vi "Lab 7.vi"() -> ()   [LabVIEW 2021]
uses:
  <vilib>/Utility/file.llb/Write Delimited Spreadsheet (string).vi
panel:
  in  "Delete User":bool
  in  "Add User":bool
  in  "Login":bool
  in  "Table Control":string[][](table)
  out "?":bool
  in  "Password:":string
  in  "Username:":string
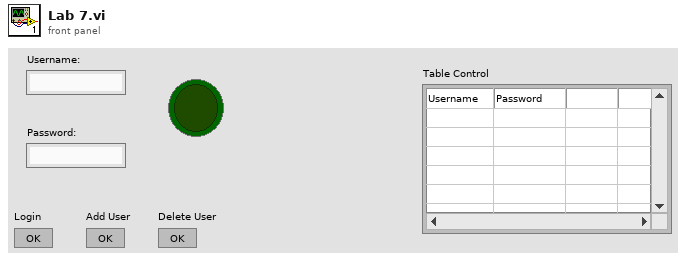
[diagram p1: front panel]
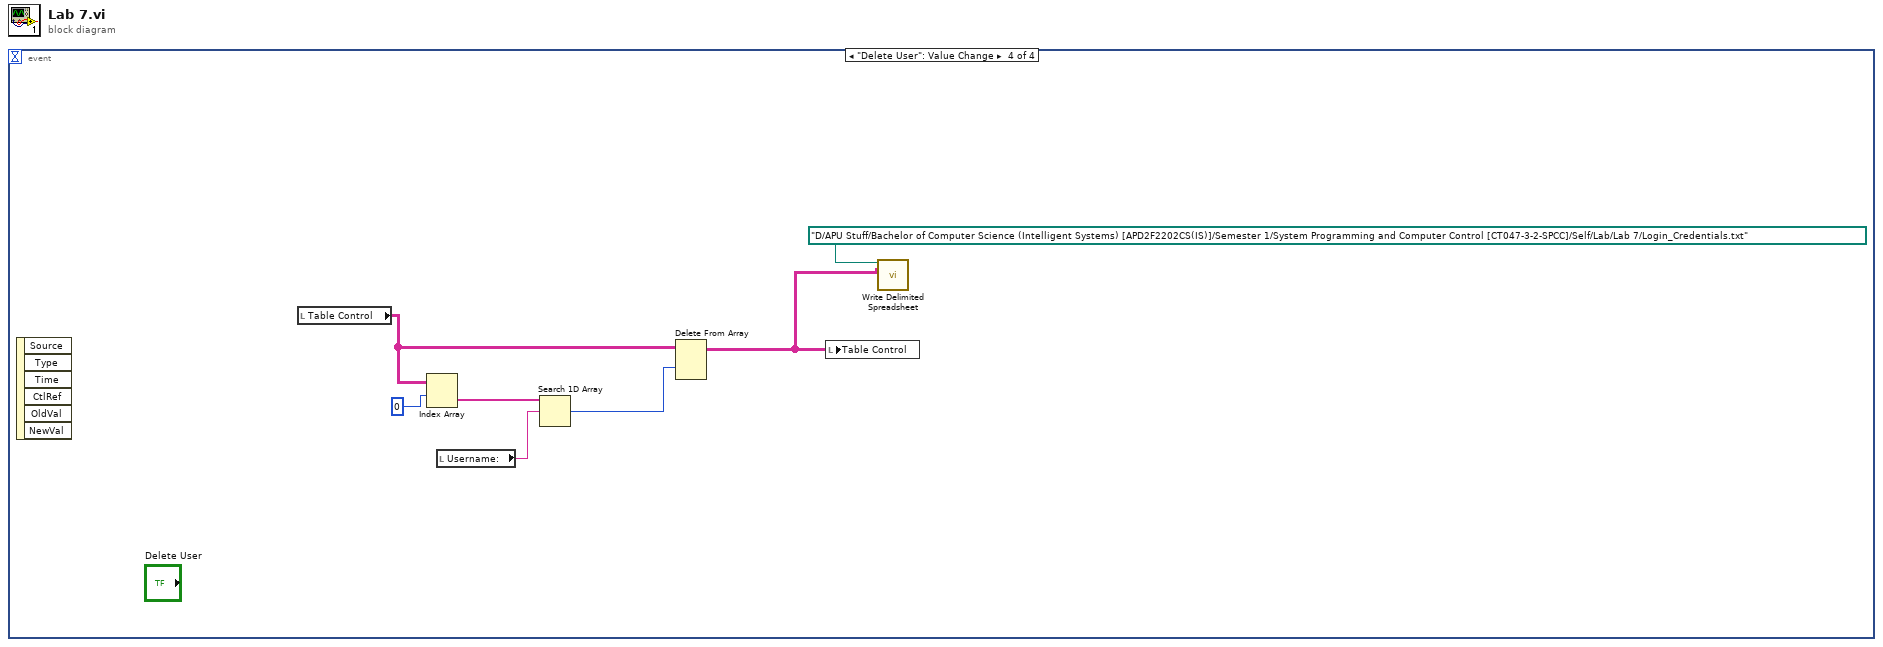
[diagram p0: block diagram]
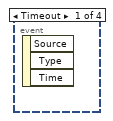
[diagram p2: hidden frame]
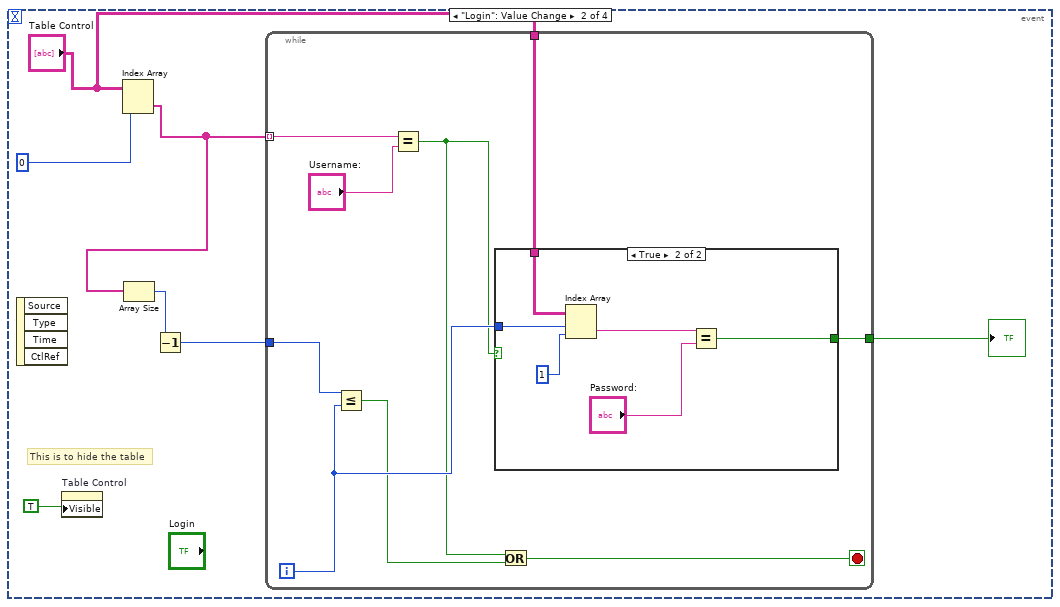
[diagram p3: hidden frame]
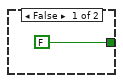
[diagram p4: hidden frame]
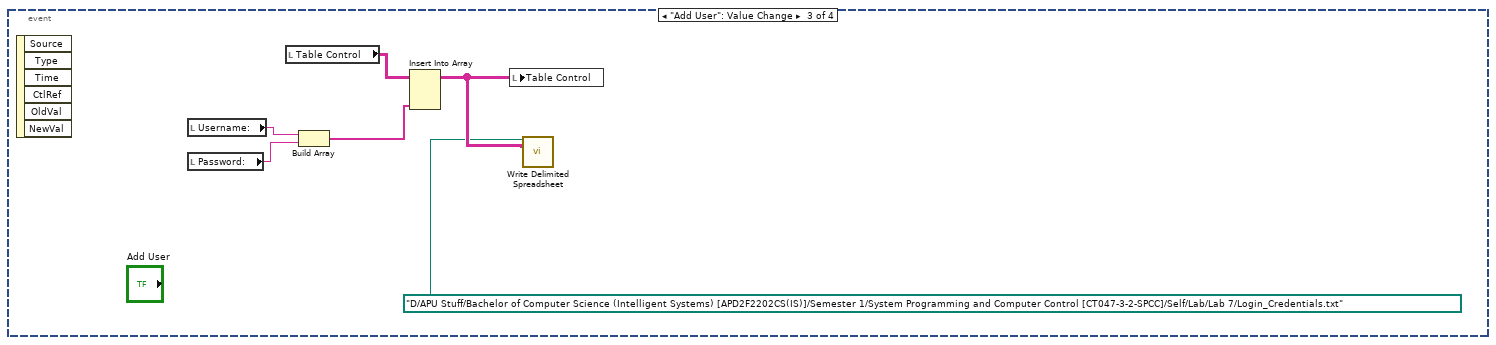
[diagram p5: hidden frame]
diagram:
  n1 = event shown="[3] \"Delete User\": Value Change" {
    selector: _ -> [_ _ _ _]
    dyn-events: _ -> [_ _ _ _]
    timeout: _ -> [_ _ _ _]
    event Timeout {
      n2 = event-data() -> ()  [unwired: 1 in, 3 out]
    }
    event "Login": Value Change {
      # "This is to hide the table"
      n3 = event-data() -> ()  [unwired: 1 in, 4 out]
      n4 = property on="Table Control" class="Tbl (strict)"("Visible"=TRUE) -> ()  [unwired: 2 in, 2 out]
      n5 = Index Array "Index Array"(array="Table Control", index (col)=0) -> (element=w5:string[])  [unwired: 1 in]
      n6 = Array Size(array=w5) -> (size(s)=w6:i32)
      n7 = Decrement(x=w6) -> (x-1=w7:i32)
      n8 = while {
        tunnel: w5 -> [w16] mode=indexing
        tunnel: "Table Control" -> [w14]
        tunnel: [w13] -> w4
        tunnel: w7 -> [w12]
        i -> [w11]
        stop <- w8 stop-if-true
        n9 = Less Or Equal?(x=w12, y=w11) -> (x <= y?=w9:bool)
        n10 = Equal?(x=w16, y="Username:") -> (x = y?=w10:bool)
        n11 = case shown="True" w10 {
          tunnel: w14 -> [_ w23]
          tunnel: [FALSE w19] -> w13
          tunnel: w11 -> [_ w18]
          frame False {
          }
          frame True {
            n12 = Index Array(array=w23, index (row)=w18, index (col)=1) -> (element=w21:string)
            n13 = Equal?(x=w21, y="Password:") -> (x = y?=w19:bool)
          }
        }
        n14 = Or(x=w10, y=w9) -> (x .or. y?=w8:bool)
      }
      "?" <- w4
    }
    event "Add User": Value Change {
      n15 = event-data() -> ()  [unwired: 1 in, 6 out]
      n16 = local read "Username:"() -> (w29:string)
      n17 = local read "Password:"() -> (w28:string)
      n18 = local read "Table Control"() -> (w27:string[][])
      n19 = Build Array "Build Array"(w29, w28) -> (w26:string[])
      n20 = Insert Into Array "Insert Into Array"(array=w27, new element=w26) -> (w25:string[][])  [unwired: 2 in]
      n21 = local write "Table Control"(w25) -> ()
      n22 = call-poly <vilib>:"Write Delimited Spreadsheet.vi"("file path (dialog if empty)"=path "D:/APU Stuff/Bachelor of Computer Science (Intelligent Systems) [APD2F2202CS(IS)]/Semester 1/System Programming and Computer Control [CT047-3-2-SPCC]/Self/Lab/Lab 7/Login_Credentials.txt", "2D data"=w25) -> ()  [unwired: 12 in, 2 out]
    }
    event "Delete User": Value Change {
      n23 = event-data() -> ()  [unwired: 1 in, 6 out]
      n24 = local read "Table Control"() -> (w33:string[][])
      n25 = Index Array "Index Array"(array=w33, index (row)=0) -> (element=w35:string[])  [unwired: 1 in]
      n26 = local read "Username:"() -> (w34:string)
      n27 = Search 1D Array(1D array=w35, element=w34) -> (index of element=w32:i32)  [unwired: 1 in]
      n28 = Delete From Array "Delete From Array"(array=w33, index (row)=w32) -> (array with subset deleted=w30:string[][])  [unwired: 2 in, 1 out]
      n29 = local write "Table Control"(w30) -> ()
      n30 = call-poly <vilib>:"Write Delimited Spreadsheet.vi"("file path (dialog if empty)"=path "D:/APU Stuff/Bachelor of Computer Science (Intelligent Systems) [APD2F2202CS(IS)]/Semester 1/System Programming and Computer Control [CT047-3-2-SPCC]/Self/Lab/Lab 7/Login_Credentials.txt", "2D data"=w30) -> ()  [unwired: 12 in, 2 out]
    }
  }
